vi "X10468 SLM Add Holo.vi"(0 "Flat On?":bool=TRUE, 2 "Holo Position":i32[](array[numeric]), 7 "Holo Array":dbl[][](array[numeric]), 11 "Flat Map":dbl[][](array[numeric])) -> (8 "Merged Flat Holo":dbl[][](array[numeric]))   [LabVIEW 2018]
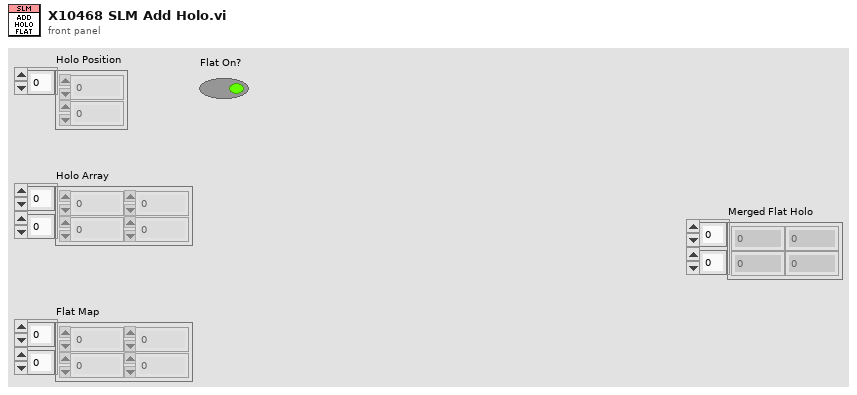
[diagram p1: front panel]
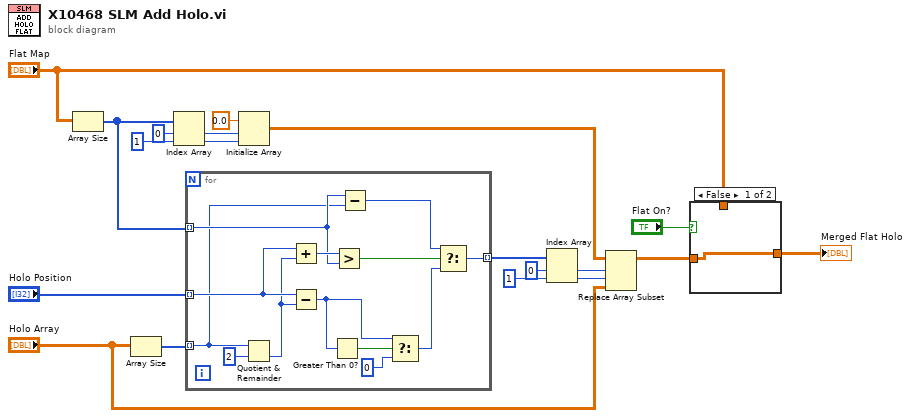
[diagram p0: block diagram]
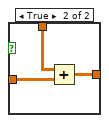
[diagram p2: hidden frame]
diagram:
  n1 = Array Size(array="Flat Map") -> (size(s)=w8:i32[])
  n2 = Array Size(array="Holo Array") -> (size(s)=w18:i32[])
  n3 = Index Array(array=w8, index #1=0 ("index"), index #2=1 ("index")) -> (element #1=w5:i32, element #2=w4:i32)
  n4 = for {
    tunnel: "Holo Position" -> [w28] mode=indexing
    tunnel: w18 -> [w21] mode=indexing
    tunnel: w8 -> [w23] mode=indexing
    tunnel: [w20] -> w17 mode=indexing
    n5 = Quotient & Remainder(x=w21, y=2) -> (floor(x/y)=w27:i32)  [unwired: 1 out]
    n6 = Add(x=w28, y=w27) -> (x+y=w26:i32)
    n7 = Subtract(x=w28, y=w27) -> (x-y=w30:i32)
    n8 = Greater Than 0?(x=w30) -> (x > 0?=w31:bool)
    n9 = Greater?(x=w26, y=w23) -> (0:w25:bool)
    n10 = Subtract(x=w23, y=w21) -> (x-y=w22:i32)
    n11 = Select(t=w30, s=w31, f=0) -> (s? t:f=w24:i32)
    n12 = Select(t=w22, s=w25, f=w24) -> (s? t:f=w20:i32)
  }
  n13 = Initialize Array(0.0 ("element"), w5, w4) -> (w2:dbl[][])
  n14 = Index Array(array=w17, index #1=0 ("index"), index #2=1 ("index")) -> (element #1=w14:i32, element #2=w13:i32)
  n15 = Replace Array Subset(array=w2, new element="Holo Array", index (row)=w14, index (col)=w13) -> (w11:dbl[][])
  n16 = case shown="False" "Flat On?" {
    tunnel: w11 -> [w33 w36]
    tunnel: "Flat Map" -> [_ w35]
    tunnel: [w33 w34] -> w9
    frame False {
    }
    frame True {
      n17 = Add(x=w35, y=w36) -> (x+y=w34:dbl[][])
    }
  }
  "Merged Flat Holo" <- w9
